vi "Exemple_Extraction_HashingVectorizer.vi"() -> ()   [LabVIEW 2020]
uses:
  Objet/6 - Datasets Transformation/6.2 - Feature extraction/HashingVectorizer/HashingVectorizer.lvclass
panel:
  in  "doc":string
  in  "X":string[][](array[string])=[["This is the first document."], ["This document is the second document."], ["And this is the third one."], ["Is this the first document?"]]
  in  "HashingVectorizer":T1={"encoding"="utf-8", "decode_error"="strict", "strip_accents"="None", "lowercase"=TRUE, "preprocessor"="None", "tokenizer"="None", "stop_words"={"Type"="None", "list"=[]}, "token_pattern"="(?u)\\b\\w\\w+\\b", "ngram_range"={"min_n"=1, "max_n"=1}, "analyzer"="word", "n_features"=1048576, "binary"=FALSE, "norm"="l2", "alternate_sign"=TRUE, "dtype"="float"}
  out "Data":T2
  out "error out":errorcluster caption="sortie d'erreur"
  in  "error in":errorcluster caption="entrée d'erreur"
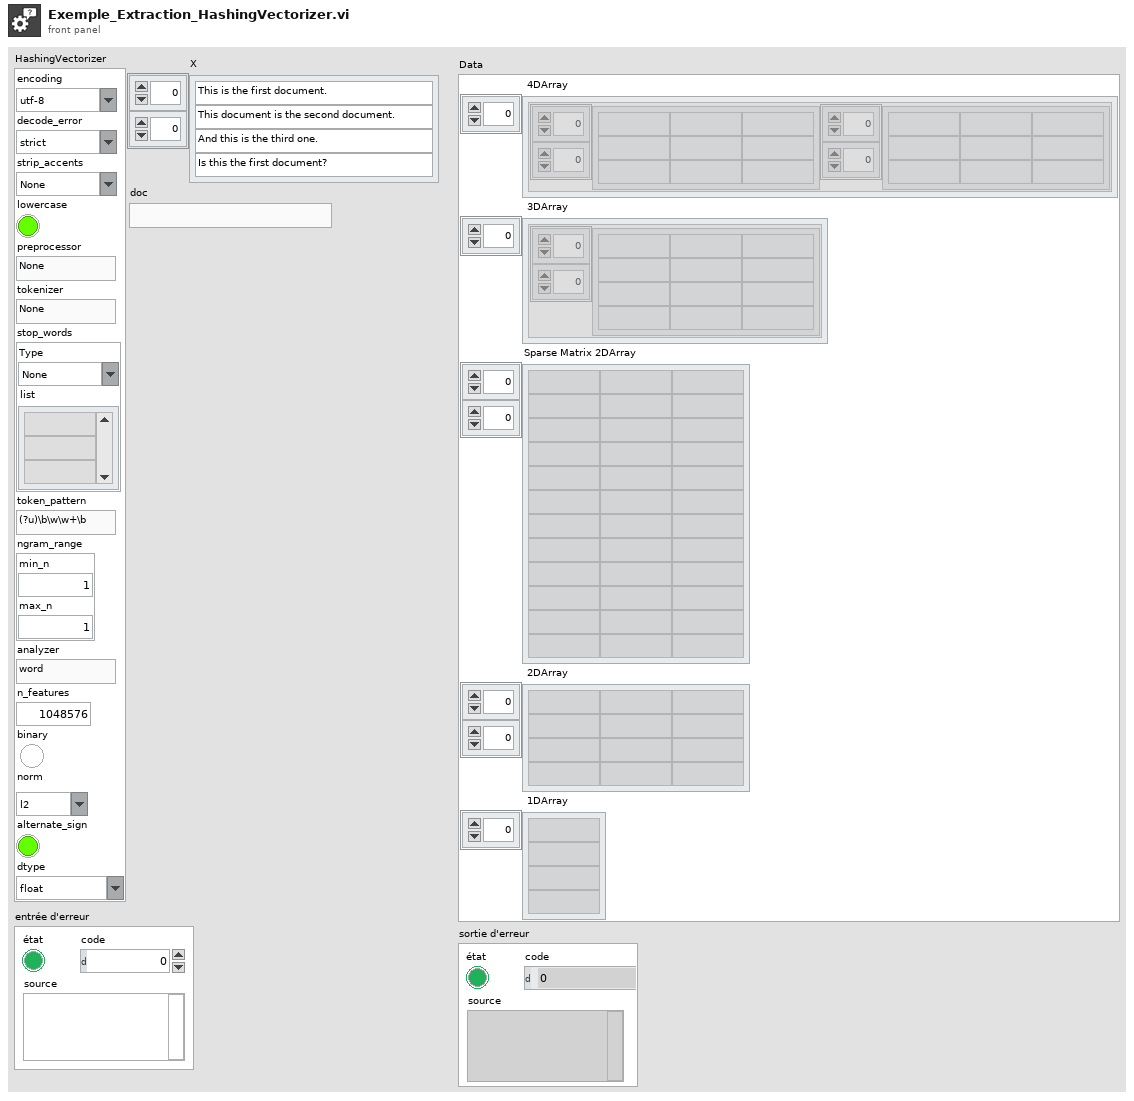
[diagram p1: front panel]
types:
  T1 = cluster{"encoding":string, "decode_error":string, "strip_accents":string, "lowercase":bool, "preprocessor":string, "tokenizer":string, "stop_words":cluster{"Type":string, "list":string[]}, "token_pattern":string, "ngram_range":cluster{"min_n":i32, "max_n":i32}, "analyzer":string, "n_features":i32, "binary":bool, "norm":string, "alternate_sign":bool, "dtype":string}
  T2 = cluster{" 4DArray":cluster{"1":string[][], "2":string[][]}[], " 3DArray":cluster{"Tableau":string[][]}[], "Sparse Matrix 2DArray":string[][], " 2DArray":string[][], " 1DArray":string[]}
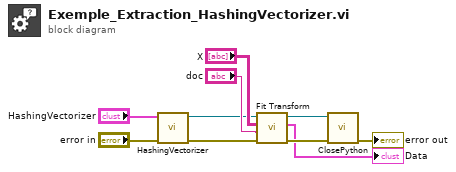
[diagram p0: block diagram]
diagram:
  n1 = call "HashingVectorizer.vi"("error in"="error in", "HashingVectorizer"="HashingVectorizer") -> ("error out"=w5:errorcluster, "HashingVectorizer.lvclass"=w6:refnum<class "HashingVectorizer.lvclass">)  [unwired: 8 in]
  n2 = call-dynamic "Fit Transform.vi"("error in (no error)"=w5, "doc"="doc", "X"="X", "HashingVectorizer.lvclass"=w6) -> ("error out"=w3:errorcluster, "Data"=→"Data":T2, "HashingVectorizer.lvclass"=w4:refnum<class "HashingVectorizer.lvclass">)  [unwired: 5 in]
  n3 = call-dynamic "ClosePython.vi"("error in (no error)"=w3, "Scikit-learn en entrée"=w4) -> ("error out"=→"error out":errorcluster)  [unwired: 8 in, 1 out]
